vi "Test Unzip File with Brackets in Name.vi"() -> ()   [LabVIEW 2019]
uses:
  <vilib>/addons/_JKI Toolkits/Caraya/classes/Assert/Assert True.vi
  source/Command-Line Zip.lvlib
  <vilib>/addons/_JKI Toolkits/Caraya/classes/Test/Test.lvclass
  <vilib>/addons/_JKI Toolkits/Caraya/classes/Assert/Assert.lvclass
panel:
  out "temp folder location":path
  out "success?":bool
  in  "Delete Temp Folder on Success?":bool=TRUE
  in  "error in":errorcluster
  out "error out":errorcluster
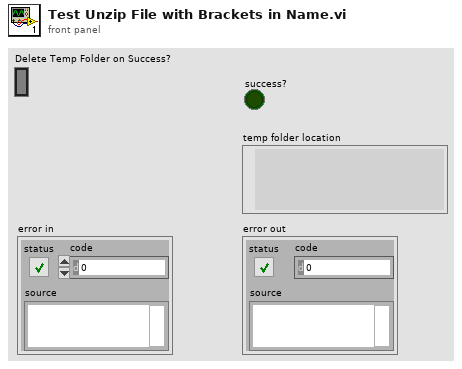
[diagram p1: front panel]
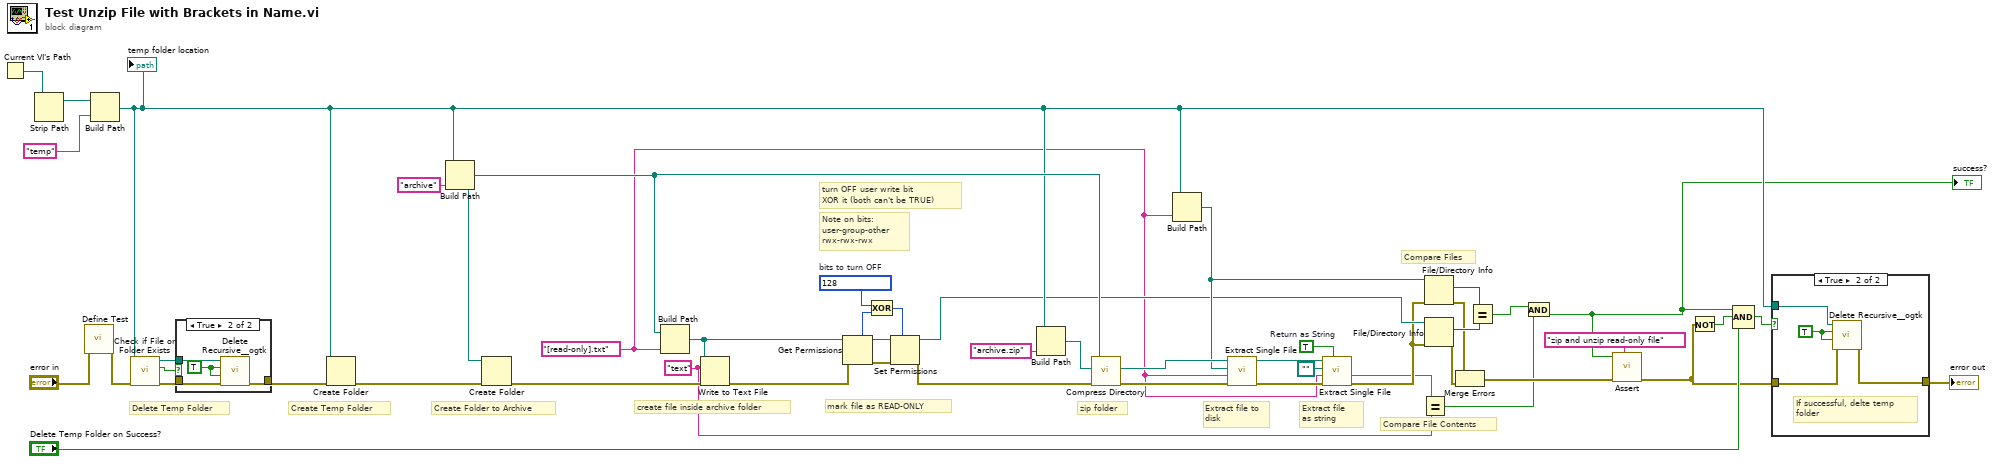
[diagram p0: block diagram]
diagram:
  w6 = TRUE  # Return as String
  w15 = i16 128  # bits to turn OFF
  w3 = "text" ("text")
  w5 = "[read-only].txt" ("name or relative path")
  # "Extract file as string"
  # "Compare File Contents"
  # "mark file as READ-ONLY"
  # "Note on bits:\nuser-group-other\nrwx-rwx-rwx"
  # "turn OFF user write bit\nXOR it (both can't be TRUE)"
  # "Extract file to disk"
  # "Compare Files"
  # "zip folder"
  # "create file inside archive folder"
  # "Create Folder to Archive"
  # "Create Temp Folder"
  # "Delete Temp Folder"
  n1 = Current VI's Path() -> (path=w50:path)
  n2 = Strip Path(path=w50) -> (stripped path=w49:path)  [unwired: 1 out]
  n3 = call <vilib>:"Define Test.vi"("error in (no error)"="error in") -> ("error out"=w24:errorcluster)  [unwired: 10 in]
  n4 = Build Path(base path=w49, name or relative path="temp") -> (appended path=w31:path)
  "temp folder location" <- w31
  n5 = call <vilib>:"Check if File or Folder Exists.vi"("error in (no error)"=w24, "path"=w31) -> ("error out"=w38:errorcluster, "file or folder exists?"=w35:bool, "dup path"=w36:path)  [unwired: 7 in]
  n6 = case shown="True" w35 {
    tunnel: w38 -> [w51 w54]
    tunnel: [w51 w55] -> w37
    tunnel: w36 -> [_ w53]
    frame False {
    }
    frame True {
      w52 = TRUE ("Recursive? (FALSE)")
      n7 = call <userlib>:"Delete Recursive__ogtk.vi"("error in (no error)"=w54, "Ignore Read-Only? (FALSE)"=w52, "Recursive? (FALSE)"=w52, "Path"=w53) -> ("error out"=w55:errorcluster)  [unwired: 6 in, 1 out]
    }
  }
  n8 = Create Folder(path (use dialog)=w31, error in=w37) -> (error out=w47:errorcluster)  [unwired: 1 in, 2 out]
  n9 = Build Path(base path=w31, name or relative path="archive") -> (appended path=w32:path)
  n10 = Create Folder(path (use dialog)=w32, error in=w47) -> (error out=w45:errorcluster)  [unwired: 1 in, 2 out]
  n11 = Build Path(base path=w32, name or relative path=w5) -> (appended path=w17:path)
  n12 = Write to Text File(file (use dialog)=w17, text=w3, error in=w45) -> (error out=w13:errorcluster)  [unwired: 1 in, 2 out]
  n13 = Get Permissions(8:w13, 11:w17) -> (0:w19:errorcluster, 3:w18:path, 5:w16:i16)  [unwired: 2 out]
  n14 = Exclusive Or(1:w16, 2:w15) -> (0:w14:i16)
  n15 = Set Permissions(7:w14, 8:w19, 11:w18) -> (0:w12:errorcluster, 3:w11:path)  [unwired: 2 in]
  n16 = Build Path(base path=w31, name or relative path="archive.zip") -> (appended path=w42:path)
  n17 = call "Compress Directory.vi"("error in (no error)"=w12, "archive name (root directory with .zip ending)"=w42, "root directory (file dialog)"=w32) -> ("error out"=w44:errorcluster, "archive name out"=w33:path)  [unwired: 6 in, 1 out]
  n18 = Build Path(base path=w31, name or relative path=w5) -> (appended path=w30:path)
  n19 = call "Extract Single File.vi"("error in (no error)"=w44, "name or relative path (\"\": use output file name)"=w5, "File output Path (extract to temp file)"=w30, "Zip File Path"=w33) -> ("error out"=w10:errorcluster, "dup Zip File Path"=w8:path)  [unwired: 4 in, 2 out]
  n20 = call "Extract Single File.vi"("Return as String (F: Extract to File)"=w6, "error in (no error)"=w10, "name or relative path (\"\": use output file name)"=w5, "File output Path (extract to temp file)"=path "", "Zip File Path"=w8) -> ("error out"=w9:errorcluster, "String"=w4:string)  [unwired: 3 in, 2 out]
  n21 = Equal?(x=w4, y=w3) -> (x = y?=w1:bool)
  n22 = File/Directory Info(path=w30, error in=w9) -> (size=w29:i64, error out=w27:errorcluster)  [unwired: 5 out]
  n23 = File/Directory Info(path=w11, error in=w9) -> (size=w28:i64, error out=w26:errorcluster)  [unwired: 5 out]
  n24 = Merge Errors(w27, w26) -> (w23:errorcluster)
  n25 = Equal?(x=w29, y=w28) -> (x = y?=w21:bool)
  n26 = And(x=w21, y=w1) -> (x .and. y?=w2:bool)
  "success?" <- w2
  n27 = call-poly <vilib>:"Assert.vi"("Label"="zip and unzip read-only file", "error in (no error)"=w23, "True?"=w2) -> ("error out"=w22:errorcluster)  [unwired: 8 in]
  n28 = Not(x=w22) -> (.not. x?=w39:bool)
  n29 = Compound Arithmetic op=AND(w2, w39, "Delete Temp Folder on Success?") -> (w40:bool)
  n30 = case shown="True" w40 {
    tunnel: [w56 w59] -> w41
    tunnel: w22 -> [w56 w58]
    tunnel: w31 -> [_ w57]
    frame False {
    }
    frame True {
      w60 = TRUE ("Recursive? (FALSE)")
      # "If successful, delte temp folder"
      n31 = call <userlib>:"Delete Recursive__ogtk.vi"("error in (no error)"=w58, "Ignore Read-Only? (FALSE)"=w60, "Recursive? (FALSE)"=w60, "Path"=w57) -> ("error out"=w59:errorcluster)  [unwired: 6 in, 1 out]
    }
  }
  "error out" <- w41
